vi "Fast Find COM Ports.vi"(8 "Error In":errorcluster) -> (0 "Error Out":errorcluster, 3 "COM Ports":string[](array[string]))   [LabVIEW 2014, in "LMH-LINX.lvlib"]
uses:
  <vilib>/MakerHub/LINX/LMH-LINX.lvlib
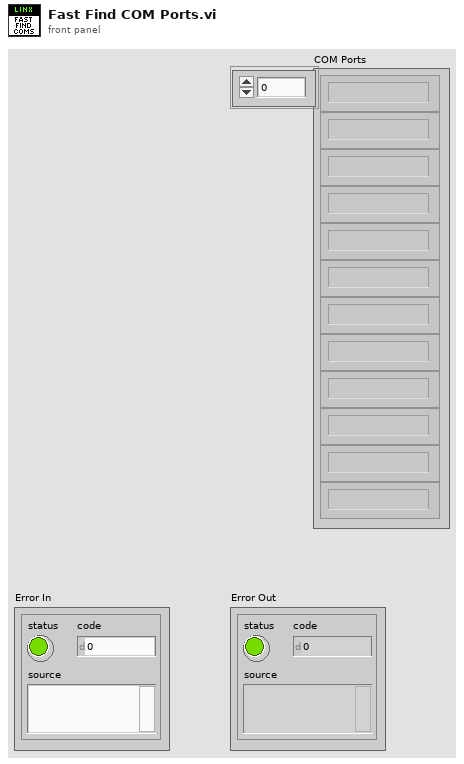
[diagram p1: front panel]
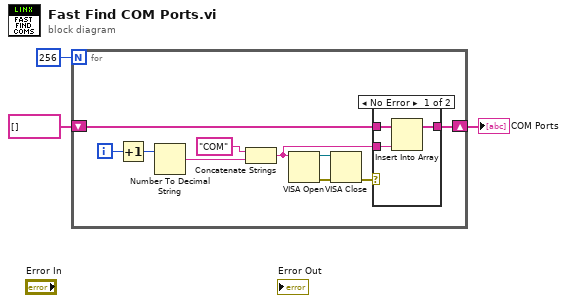
[diagram p0: block diagram]
diagram:
  n1 = for {
    N: 256 -> [_]
    shift-right: [w5] -> w2
    shift-left: string[] [] -> [w6]
    i -> [w9]
    n2 = Increment(x=w9) -> (x+1=w8:i32)
    n3 = Number To Decimal String(number=w8) -> (decimal integer string=w10:string)  [unwired: 1 in]
    n4 = Concatenate Strings("COM", w10) -> (w4:string)
    n5 = VISA Open(VISA resource name=w4) -> (VISA resource name=w12:refnum<visa-resource-name>, error out=w13:errorcluster)  [unwired: 4 in]
    n6 = VISA Close(VISA resource name=w12, error in (no error)=w13) -> (error out=w7:errorcluster)
    n7 = case shown="No Error" w7 {
      tunnel: w6 -> [w16 w17]
      tunnel: [w15 w17] -> w5
      tunnel: w4 -> [w14 _]
      frame No Error {
        n8 = Insert Into Array(array=w16, new element=w14) -> (w15:string[])  [unwired: 1 in]
      }
      frame Error {
      }
    }
  }
  "COM Ports" <- w2
